vi "Read Tcp.vi"(8 "error in (no error)":errorcluster, 11 "Cli in":refnum<class "Cli.lvclass">) -> (0 "error out":errorcluster, 2 "Tcp":refnum<class "Message Enqueuer.lvclass">, 3 "Cli out":refnum<class "Cli.lvclass">)   [LabVIEW 2022 SP3, in "Cli.lvlib" / "Cli.lvclass"]
uses:
  Cli.lvclass
  Cli.lvclass/Cli.ctl
  <vilib>/ActorFramework/Message Enqueuer/Message Enqueuer.lvclass
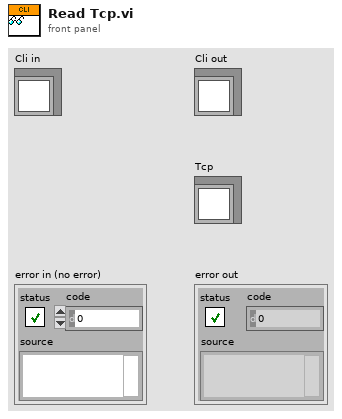
[diagram p1: front panel]
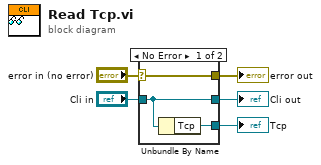
[diagram p0: block diagram]
diagram:
  n1 = case shown="No Error" "error in (no error)" {
    selector: "error in (no error)" -> [w8 w9]
    tunnel: [w8 w9] -> w4
    tunnel: [w7 w10] -> w2
    tunnel: "Cli in" -> [w7 w10]
    tunnel: [w6 _] -> w1
    frame No Error {
      n2 = Unbundle By Name(w7) -> ("Tcp"=w6:refnum<class "Message Enqueuer.lvclass">)
    }
    frame Error {
    }
  }
  "error out" <- w4
  "Cli out" <- w2
  "Tcp" <- w1
